vi "connect.vi"(0 "PI_Piezo.lvclass (in)":refnum<class "PI_Piezo.lvclass">, 11 "error in":errorcluster) -> (4 "PI_Piezo.lvclass":refnum<class "PI_Piezo.lvclass">, 15 "error out":errorcluster)   [LabVIEW 2013, in "PI_Piezo.lvclass"]
doc: "This VI demonstrates how to initialize an E-816 system with more than one axis, how to move all connected axes and how to query for the position value. \n\nIn this example the E-816 is connected through USB. The Serial No. of the system to command is not known, so the \"Search for controllers\" control is left TRUE. The VI runs E816_Configuration_Setup.vi with specified settings, moves the connected axes relative to their current position, waits for the movement to finish and reads the position of the axes and the error status of the controller. Instead of calling the corresponding command VIs, it uses \"Split multiple axes command.vi\" which sends the chosen commands for the given axes one after another and returns the answer array (if any). The diagram shows how to combine the driver VIs for these tasks. \n\nFor an example of how to command a single axis E-816 system connected through RS-232 see E816_Sample_ Application_1.vi\n\nWarning: Before running this VI, modify the interface settings on the block diagram to reflect your configuration. The predefined settings provided with the VI probably do not match your system."
uses:
  PI_Piezo.lvclass
  PI_Piezo.lvclass/PI_Piezo.ctl
panel:
  # "This VI demonstrates how to initialize an E-816 system with more than one axis, how to move all connected axes and how to query\nfor the position value. The VI runs E816_Configuration_Setup.vi with specified settings, moves the connected axes relative to their \ncurrent position and reads the position. Instead of calling the corresponding command VIs, it uses \"Split multiple axes command.vi\"\nwhich sends the chosen commands for the given axes one after another and returns the answer array (if any). The diagram shows\nhow to combine the driver VIs for these tasks. \n\nWarning: Before running this VI, modify the interface settings on the block diagram to reflect your configuration. The predefined \n                 settings provided with the VI probably do not match your system."
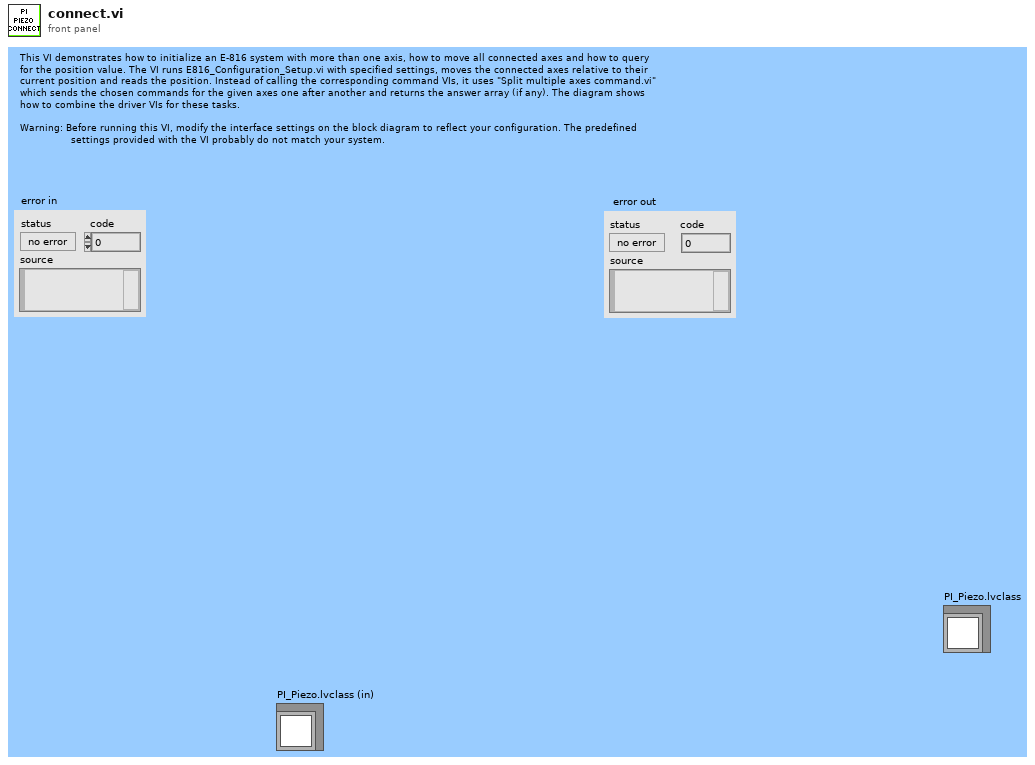
[diagram p1: front panel]
types:
  T1 = typedef "PI_Piezo.lvclass/settings.ctl" = cluster{"Enable":bool, "Array of Piezo Controllers":T2[]}
  T2 = typedef "PI_Piezo.lvclass/piezo_controller.ctl" = cluster{"Enable":bool, "Serial No.":string, "Array of Piezo Channels":T3[]}
  T3 = typedef "PI_Piezo.lvclass/piezo_channel.ctl" = cluster{"Servo":bool, "Set Position":dbl}
  T4 = enum16{"DCO", "DCO?", "MOV", "MOV?", "MVR", "ONT?", "OVF?", "POS?", "RST", "SVA", "SVA?", "SVO", "SVO?", "SVR", "VOL?", "GWait"}
  T5 = cluster{"Axis":string, "Servo":bool, "Position":dbl}
  T6 = cluster{"Identification":string, "SN out":string, cluster{"Axis":string, "Servo":bool, "Position":dbl}[]}
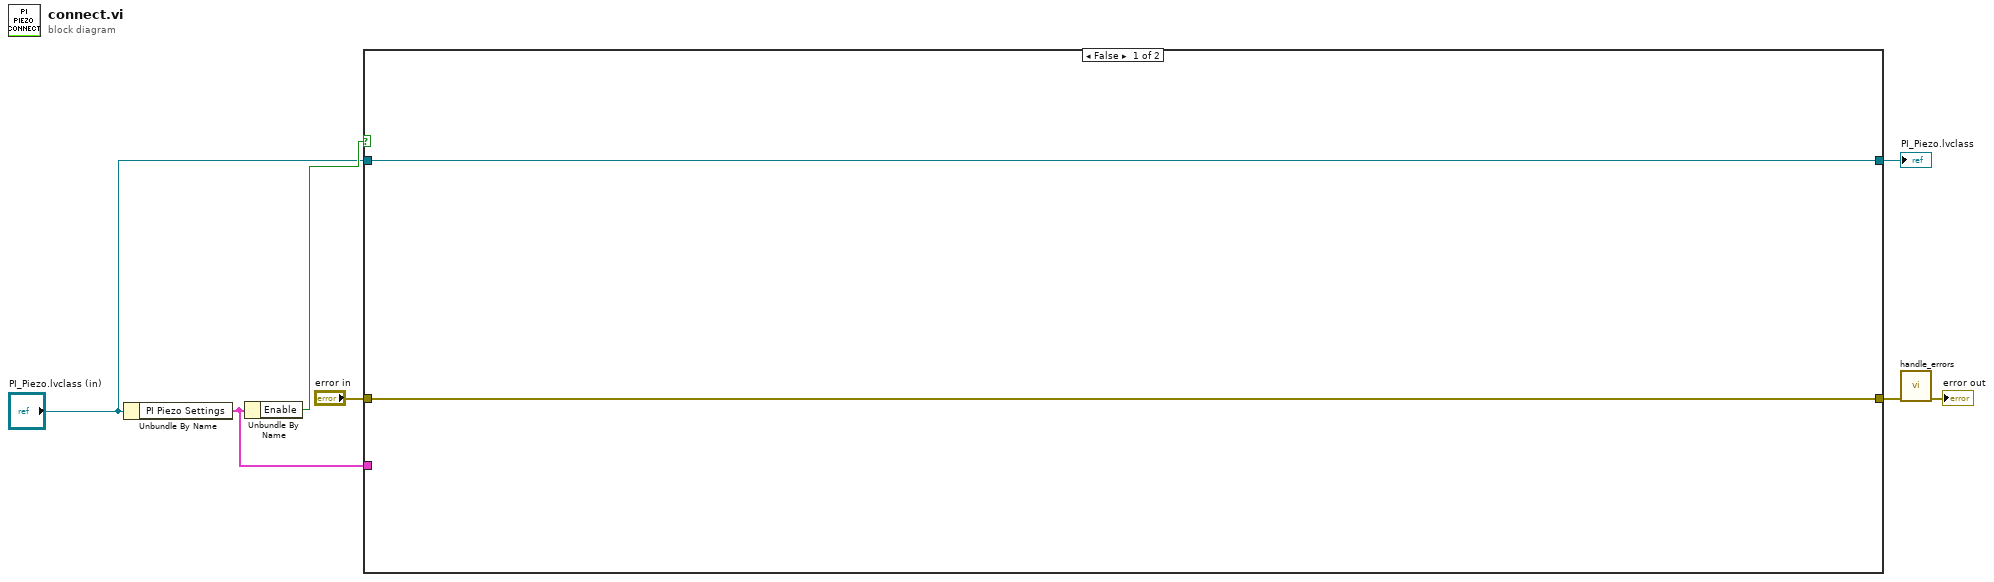
[diagram p0: block diagram]
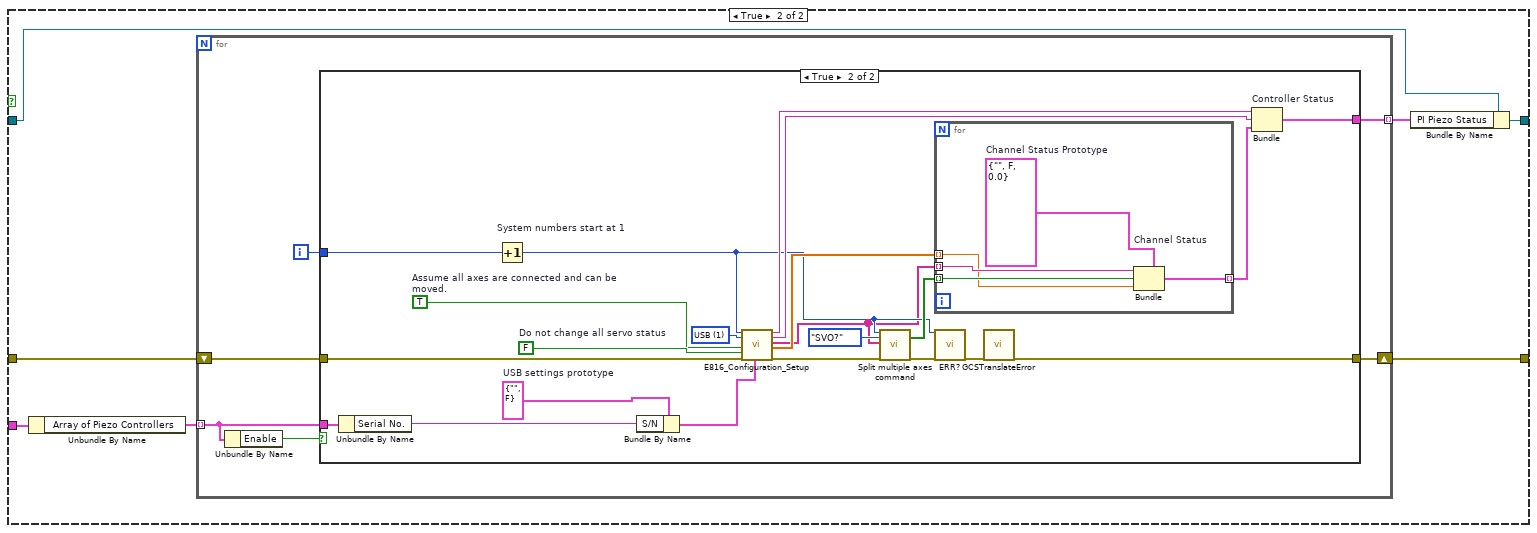
[diagram p2: hidden frame]
diagram:
  n1 = Unbundle By Name("PI_Piezo.lvclass (in)") -> ("PI Piezo Settings"=w3:T1)
  n2 = Unbundle By Name(w3) -> ("Enable"=w5:bool)
  n3 = case shown="False" w5 {
    tunnel: w3 -> [_ w16]
    tunnel: "error in" -> [w9 w14]
    tunnel: [w9 w10] -> w6
    tunnel: [w8 w13] -> w2
    tunnel: "PI_Piezo.lvclass (in)" -> [w8 w12]
    frame False {
    }
    frame True {
      n4 = Unbundle By Name(w16) -> ("Array of Piezo Controllers"=w15:T2[])
      n5 = for {
        tunnel: w15 -> [w20] mode=indexing
        shift-right: [w18] -> w10
        shift-left: w14 -> [w19]
        tunnel: [w17] -> w11 mode=indexing
        i -> [w21]
        n6 = Unbundle By Name(w20) -> ("Enable"=w22:bool)
        n7 = case shown="True" w22 {
          tunnel: w21 -> [_ w45]
          tunnel: w20 -> [_ w43]
          tunnel: w19 -> [w23 w38]
          tunnel: [w23 w32] -> w18
          tunnel: [_ w35] -> w17
          frame False {
          }
          frame True {
            w34 = TRUE  # Assume all axes are connected and can be moved.
            w39 = FALSE  # Do not change all servo status
            w41 = cluster{"S/N":string, "USB Search?":bool} {"S/N"="", "USB Search?"=FALSE}  # USB settings prototype
            w44 = u16 1 items=["RS232", "USB"] ("Interface")
            n8 = Unbundle By Name(w43) -> ("Serial No."=w42:string)
            n9 = Increment "System numbers start at 1"(x=w45) -> (x+1=w27:i32)
            n10 = Bundle By Name(cluster=w41, "S/N"=w42) -> (w40:cluster{"S/N":string, "USB Search?":bool})
            n11 = call "E816_Configuration_Setup.vi"("System no."=w27, "Interface"=w44, "All axes?"=w34, "Change servo \nstatus to ON?"=w39, "error in"=w38, "USB settings"=w40) -> ("Identification"=w37:string, "SN out"=w36:string, "Conn. Axes"=w26:string[], "Position"=w30:dbl[], "error out"=w25:errorcluster)  [unwired: 9 in]
            n12 = call "Split multiple axes command.vi"("System no."=w27, "Command"=T4."SVO?", "Axes to command"=w26, "error in"=w25) -> ("Bool. values out"=w28:bool[], "error out"=w24:errorcluster)  [unwired: 13 in, 1 out]
            n13 = for {
              tunnel: w28 -> [w50] mode=indexing
              tunnel: [w49] -> w31 mode=indexing
              tunnel: w26 -> [w48] mode=indexing
              tunnel: w30 -> [w46] mode=indexing
              w47 = T5 {"Axis"="", "Servo"=FALSE, "Position"=0.0}  # Channel Status Prototype
              n14 = Bundle "Channel Status"(cluster=w47, "Axis"=w48, "Servo"=w50, "Position"=w46) -> (w49:T5)
            }
            n15 = call "ERR?.vi"("System no."=w27, "error in"=w24) -> ("error out"=w33:errorcluster)  [unwired: 16 in, 1 out]
            n16 = call "GCSTranslateError.vi"("error in"=w33) -> ("error out"=w32:errorcluster)  [unwired: 16 in, 2 out]
            n17 = Bundle "Controller Status"("Identification"=w37, "SN out"=w36, w31) -> (w35:T6)  [unwired: 1 in]
          }
        }
      }
      n18 = Bundle By Name(cluster=w12, "PI Piezo Status"=w11) -> (w13:refnum<class "PI_Piezo.lvclass">)
    }
  }
  "PI_Piezo.lvclass" <- w2
  n19 = call "handle_errors.vi"("error in (no error)"=w6) -> ("error out"=→"error out":errorcluster)  [unwired: 10 in]
